vi "FTW-Actor-Initialized.vi"(0 "FTW Actor Instance":refnum<class "FTW-ActorInstance.lvclass">, 5 "Initialized Response":string, 11 "error in":errorcluster) -> (4 "FTW Actor Instance out":refnum<class "FTW-ActorInstance.lvclass">, 15 "error out":errorcluster)   [LabVIEW 2012, in "FTW-Actor.lvlib" / "FTW-ActorInstance.lvclass"]
uses:
  FTW-ActorInstance.lvclass
  FTW-Actor-FrameworkEvent.ctl
  FTW-ActorInstance.lvclass/FTW-ActorInstance.ctl
  Core/src/Time/FTW-Time-DisplayFormat-Timestamp.ctl
  Endpoint/FTW-Endpoint-Type.ctl
  Endpoint/FTW-Endpoint.lvclass
panel:
  # "Inputs"
  # "Outputs"
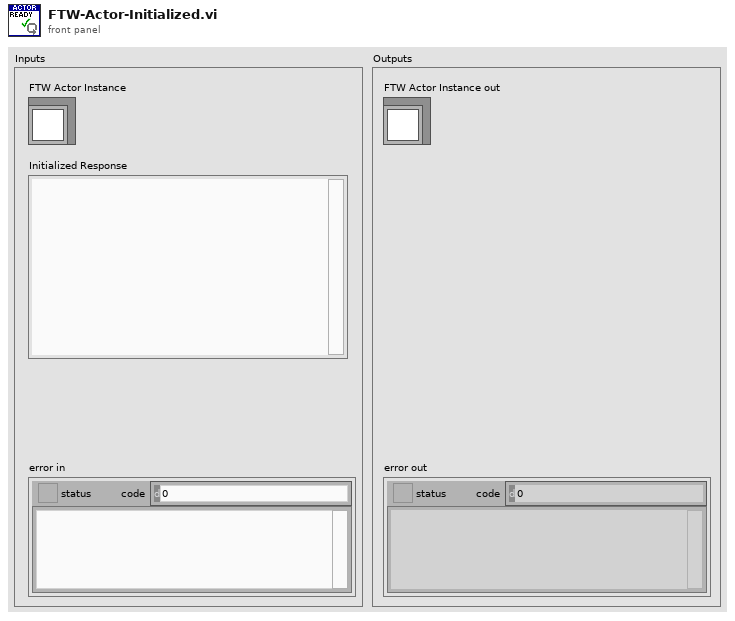
[diagram p1: front panel]
types:
  T1 = typedef "FTW-Actor.lvlib/FTW-ActorInstance.lvclass/FTW-Actor-FrameworkEvent.ctl" = enum16{"Instance Initializing", "Instance Initialized", "Instance Job", "Instance Handle Request", "Instance Shutting Down", "Instance Destroyed"}
  T2 = typedef "FTW-Time-DisplayFormat-Timestamp.ctl" = enum16{"YYYY-MM-DDT00:00:00.000Z (ISO-8601)", "YYYY-MM-DDT00-00-00Z (Simple ISO-8601)", "YYYY-MM-DD"}
  T3 = typedef "FTW-Actor.lvlib/FTW-Endpoint.lvclass/FTW-Endpoint-Type.ctl" = enum32{"Server", "Client", "Publisher", "Subscriber", "Pipeline Producer", "Pipeline Consumer", "Surveyor", "Respondent", "Exclusive Pair", "Bus"}
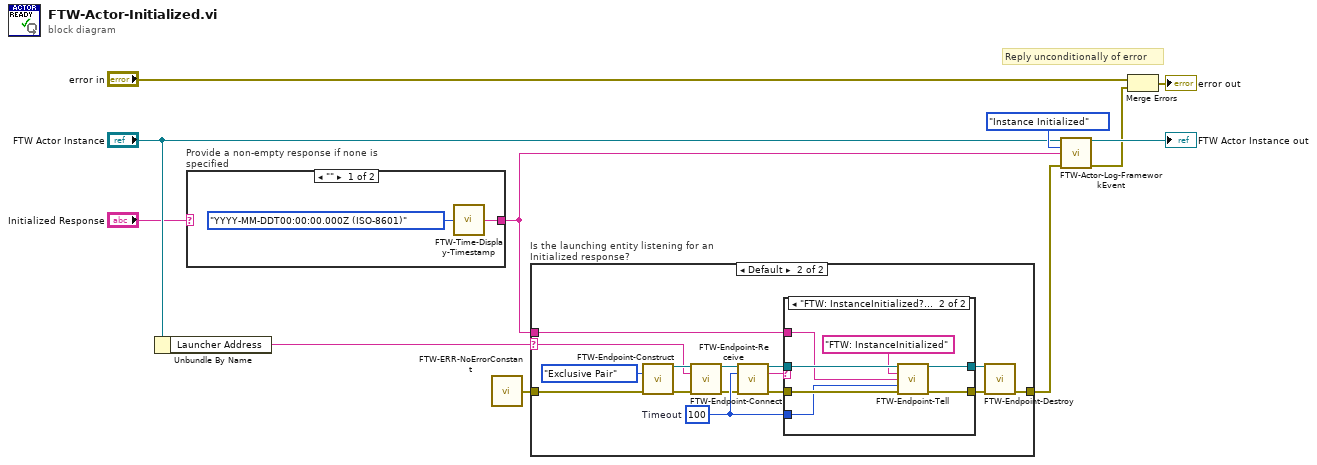
[diagram p0: block diagram]
diagram:
  # "Reply unconditionally of error"
  n1 = Unbundle By Name("FTW Actor Instance") -> ("Launcher Address"=w7:string)
  n2 = case "Provide a non-empty response if none is specified" shown="\"\"" "Initialized Response" {
    selector: "Initialized Response" -> [_ w14]
    tunnel: [w13 w14] -> w5
    frame "" {
      n3 = call "FTW-Time-Display-Timestamp.vi"("Format"=FTW-Time-DisplayFormat-Timestamp."YYYY-MM-DDT00:00:00.000Z (ISO-8601)") -> ("Formatted Timestamp"=w13:string)  [unwired: 3 in]
    }
    frame Default {
    }
  }
  n4 = call "FTW-ERR-NoErrorConstant.vi"() -> ("no error"=w4:errorcluster)
  n5 = case "Is the launching entity listening for an Initialized response?" shown="Default" w7 {
    selector: w7 -> [_ w20]
    tunnel: w5 -> [_ w28]
    tunnel: [w15 w25] -> w8
    tunnel: w4 -> [w15 w19]
    frame "" {
    }
    frame Default {
      w24 = 100  # Timeout
      n6 = call "FTW-Endpoint-Construct.vi"("Socket Type"=FTW-Endpoint-Type."Exclusive Pair", "error in"=w19) -> ("FTW Socket"=w22:refnum<class "FTW-Endpoint.lvclass">, "error out"=w21:errorcluster)  [unwired: 12 in]
      n7 = call-dynamic "FTW-Endpoint-Connect.vi"("FTW Socket"=w22, "Remote Address"=w20, "error in"=w21) -> ("FTW Socket out"=w18:refnum<class "FTW-Endpoint.lvclass">, "error out"=w17:errorcluster)  [unwired: 11 in]
      n8 = call-dynamic "FTW-Endpoint-Receive.vi"("FTW Endpoint"=w18, "Timeout"=w24, "error in"=w17) -> ("FTW Endpoint out"=w27:refnum<class "FTW-Endpoint.lvclass">, "Message Header"=w16:string, "error out"=w30:errorcluster)  [unwired: 8 in, 2 out]
      n9 = case shown="\"FTW: InstanceInitialized?\"" w16 {
        tunnel: w30 -> [w32 w39]
        tunnel: [w31 w38] -> w29
        tunnel: w28 -> [_ w33]
        tunnel: w27 -> [w31 w37]
        tunnel: [w32 w36] -> w26
        tunnel: w24 -> [_ w35]
        frame Default {
        }
        frame "FTW: InstanceInitialized?" {
          n10 = call-dynamic "FTW-Endpoint-Tell.vi"("FTW Socket"=w37, "Message Header"="FTW: InstanceInitialized", "Message Body"=w33, "Timeout"=w35, "error in"=w39) -> ("FTW Socket out"=w38:refnum<class "FTW-Endpoint.lvclass">, "error out"=w36:errorcluster)  [unwired: 8 in, 1 out]
        }
      }
      n11 = call-dynamic "FTW-Endpoint-Destroy.vi"("FTW Socket"=w29, "error in"=w26) -> ("error out"=w25:errorcluster)  [unwired: 13 in]
    }
  }
  n12 = call "FTW-Actor-Log-FrameworkEvent.vi"("FTW Actor Instance"="FTW Actor Instance", "Framework Event"=FTW-Actor-FrameworkEvent."Instance Initialized", "Event Data"=w5, "error in"=w8) -> ("FTW Actor Instance out"=→"FTW Actor Instance out":refnum<class "FTW-ActorInstance.lvclass">, "error out"=w3:errorcluster)  [unwired: 10 in]
  n13 = Merge Errors("error in", w3) -> (→"error out":errorcluster)
